vi "LockinDAQ.Start.vi"(8 "error in":errorcluster, 11 "LockinDAQ":refnum<class "LockinDAQ.lvclass">) -> (0 "error out":errorcluster, 3 "LockinDAQ out":refnum<class "LockinDAQ.lvclass">)   [LabVIEW 2016, in "LockinDAQ.lvclass"]
uses:
  LockinDAQ.lvclass
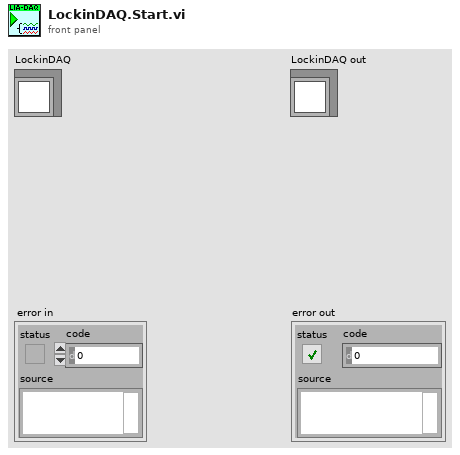
[diagram p1: front panel]
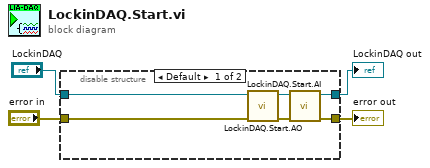
[diagram p0: block diagram]
diagram:
  n1 = disable-structure shown="Default" {
    disable-tunnel: "LockinDAQ" -> [w6 w12]
    disable-tunnel: "error in" -> [w5 w11]
    disable-tunnel: [w8 w12] -> w2
    disable-tunnel: [w7 w11] -> w1
    frame condition #0 (active) {
      n2 = call "LockinDAQ.Start.AO.vi"("error in (no error)"=w5, "LockinDAQ"=w6) -> ("error out"=w10:errorcluster, "LockinDAQ out"=w9:refnum<class "LockinDAQ.lvclass">)  [unwired: 8 in]
      n3 = call "LockinDAQ.Start.AI.vi"("error in (no error)"=w10, "LockinDAQ"=w9) -> ("error out"=w7:errorcluster, "LockinDAQ out"=w8:refnum<class "LockinDAQ.lvclass">)  [unwired: 6 in]
    }
    frame condition #1 {
    }
  }
  "error out" <- w1
  "LockinDAQ out" <- w2
